vi "RTM - Remove Packets Dependency.vi"(8 "error in (no error)":errorcluster, 9 "Menu hierarchy in":string[](array[string]), 11 "Node Ptr":u64 format="%.0x") -> (0 "error out":errorcluster, 1 "Menu hierarchy out":string[](array[string]), 3 "Action":T1)   [LabVIEW 2015, in "UDP-Custom-Device System Explorer.lvlib"]
uses:
  UDP-Custom-Device System Explorer.lvlib
  <vilib>/NI Veristand/Custom Device API/Custom Device RTM Dependency.ctl
  Shared/Constants.vi
  <vilib>/NI Veristand/Custom Device API/Get Item Property (String Array).vi
  <vilib>/NI VeriStand/Custom Device API/Custom Device API.lvlib
  Shared/UDP-Custom-Device Shared.lvlib
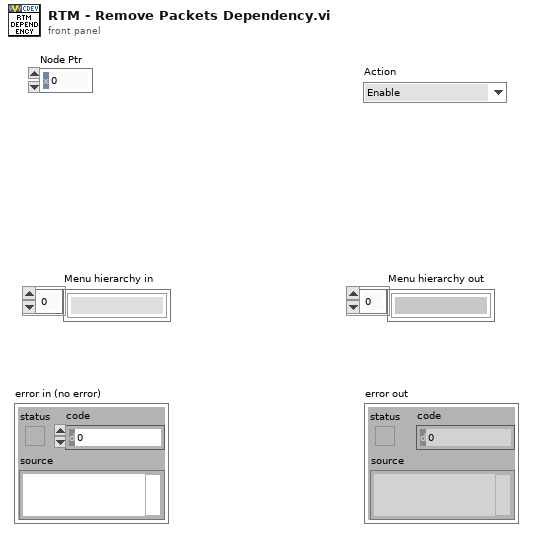
[diagram p1: front panel]
types:
  T1 = typedef "Custom Device API.lvlib/Custom Device RTM Dependency.ctl" = enum16{"Enable", "Disable", "Hide"}
  T2 = typedef "Custom Device API.lvlib/Custom Device Item Ref.ctl" = u64
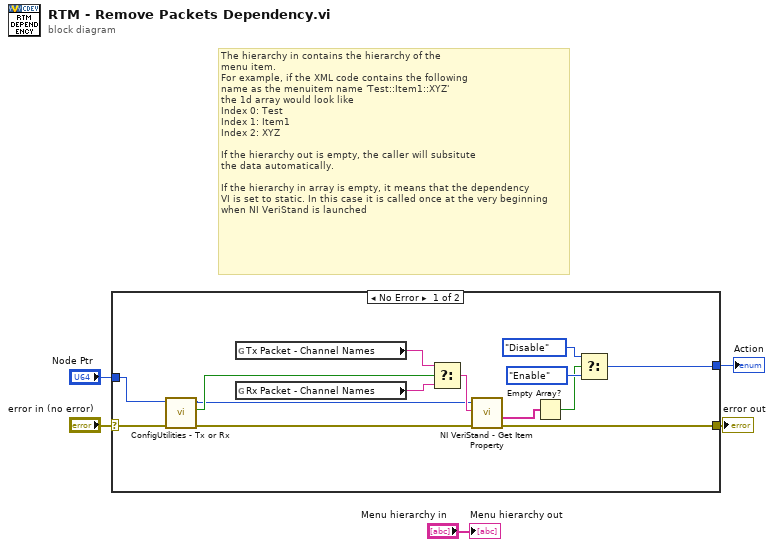
[diagram p0: block diagram]
diagram:
  # "The hierarchy in contains the hierarchy of the\nmenu item.\nFor example, if the XML code contains the following\nname as the menuitem name 'Test::Item1::XYZ'\nthe 1d array would look like\nIndex 0: Test\nIndex 1: Item1\nIndex 2: XYZ\n\nIf the hierarchy out is empty, the caller will subsitute\nthe data automatically.\n\nIf the hierarchy in array is empty, it means that the dependency\nVI is set to static. In this case it is called once at the very beginning\nwhen NI VeriStand is launched"
  n1 = case shown="No Error" "error in (no error)" {
    selector: "error in (no error)" -> [w10 w20]
    tunnel: "Node Ptr" -> [w9 _]
    tunnel: [w19 _] -> w3
    tunnel: [w18 w20] -> w1
    frame No Error {
      n2 = call "ConfigUtilities - Tx or Rx.vi"("error in (no error)"=w10, "Item Ref in"=w9) -> ("error out"=w6:errorcluster, "Tx?"=w8:bool, "Item Ref out"=w7:T2)  [unwired: 7 in]
      n3 = global read "Constants.vi" "Tx Packet - Channel Names"() -> (w15:string)
      n4 = global read "Constants.vi" "Rx Packet - Channel Names"() -> (w14:string)
      n5 = Select(t=w15, s=w8, f=w14) -> (s? t:f=w11:string)
      n6 = call-poly <vilib>:"NI VeriStand - Get Item Property.vi"("error in (no error)"=w6, "Property Name"=w11, "Item Ref in"=w7) -> ("error out"=w18:errorcluster, "Value"=w12:string[])  [unwired: 5 in, 2 out]
      n7 = Empty Array?(array=w12) -> (empty?=w13:bool)
      n8 = Select(t=Custom_Device_RTM_Dependency."Disable" ("Action"), s=w13, f=Custom_Device_RTM_Dependency."Enable" ("Action")) -> (s? t:f=w19:T1)
    }
    frame Error {
    }
  }
  "error out" <- w1
  "Action" <- w3
  "Menu hierarchy out" <- "Menu hierarchy in"
